vi "Actor Core.vi"(8 "error in":errorcluster, 11 "Nested in":refnum<class "UI_Top.lvclass">) -> (0 "error out":errorcluster, 3 "Actor out":refnum<class "Actor.lvclass">)   [LabVIEW 2021, in "UI_Top.lvclass"]
doc: "(<B>Filename</B>: Actor Framework.lvlib:Actor.lvclass:Actor Core.vi)\n\nReceives messages to the actor, reacts to them, and initiates any error handling that may shut the actor down.\n\nDescendant classes may override this VI to append parallel tasks for the actor to complete while it handles messages. Overrides use the Call Parent Method node."
uses:
  UI_Top.lvclass
  C:/Program Files (x86)/National Instruments/LabVIEW 2021/user.lib/John_Lib/AbstractActorTemplate/AbstractActorTemplate/UIActorTop.lvclass
  C:/Program Files (x86)/National Instruments/LabVIEW 2021/vi.lib/ActorFramework/Actor/Actor.lvclass
  <vilib>/ActorFramework/Actor/Actor.lvclass
  <userlib>/John_Lib/Control/Panel State.ctl
  UI_Top.lvclass/UI_Top.ctl
  <vilib>/ActorFramework/Actor/Actor.lvclass/Actor.ctl
  <vilib>/ActorFramework/Message Enqueuer/Message Enqueuer.lvclass/Message Enqueuer.ctl
  <userlib>/John_Lib/AbstractActorTemplate/UIActorTop Messages/UI Front Panel State Msg/UI Front Panel State Msg.lvclass/UI Front Panel State Msg.ctl
  <vilib>/ActorFramework/Message Enqueuer/Init from Existing Queue.vi
  <vilib>/ActorFramework/Message Enqueuer/Enqueue.vi
  <userlib>/John_Lib/AbstractActorTemplate/UIActorTop Messages/UI Front Panel State Msg/UI Front Panel State Msg.lvclass
  C:/Program Files (x86)/National Instruments/LabVIEW 2021/vi.lib/ActorFramework/Message/Message.lvclass
  <vilib>/ActorFramework/Stop Msg/Stop Msg.lvclass
  <vilib>/ActorFramework/Message Priority Queue/Priority Enqueue.vi
  <vilib>/ActorFramework/Message Enqueuer/Message Enqueuer.lvclass
  <userlib>/John_Lib/AbstractActorTemplate/AbstractActorTemplate/UIActorTop.lvclass
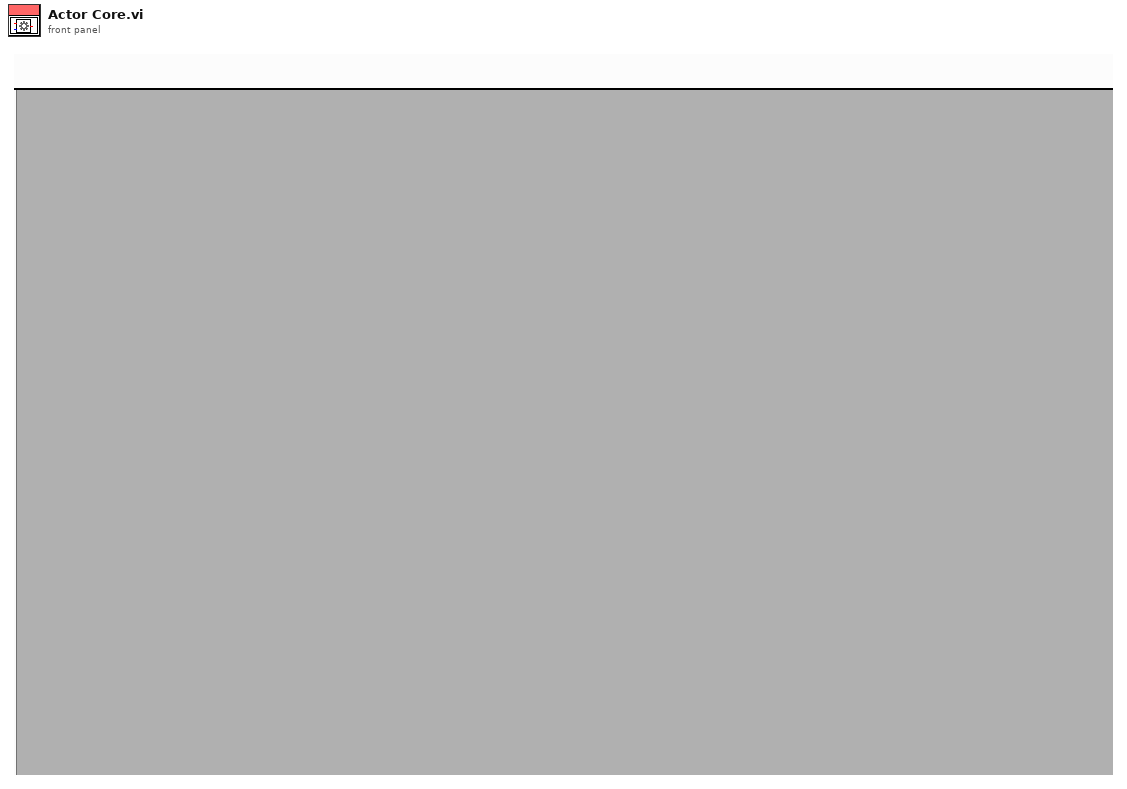
[diagram p1: front panel]
types:
  T1 = typedef "Panel State.ctl" = string
  T2 = typedef "sizeaction.ctl" = enum32{"Minimized", "Maximized", "Resized"}
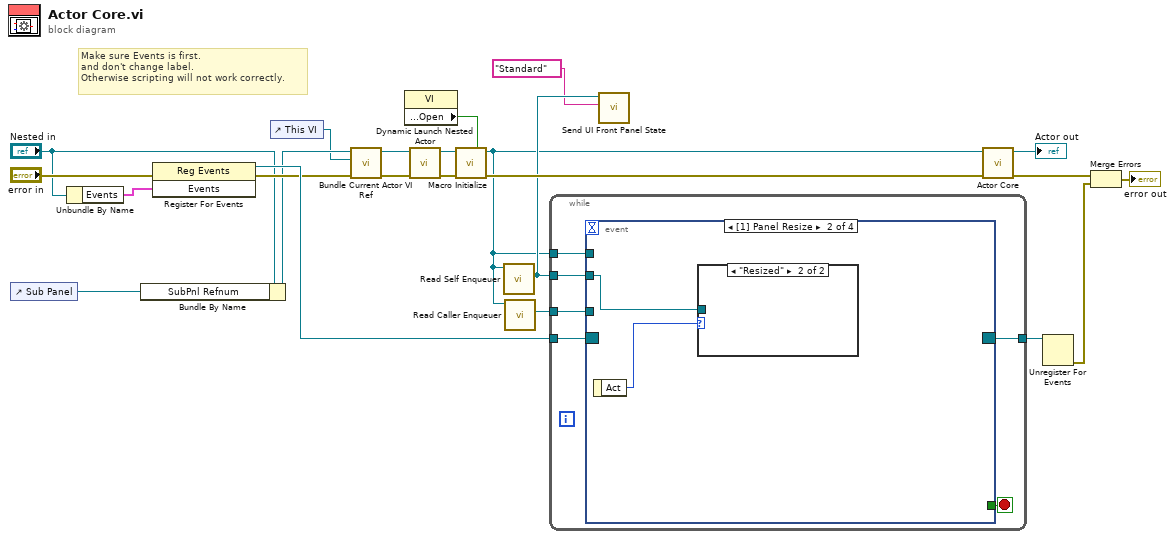
[diagram p0: block diagram]
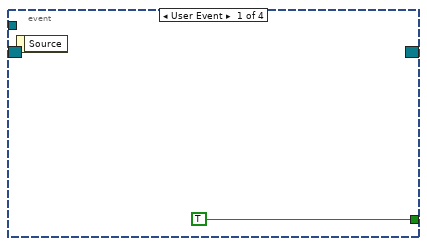
[diagram p2: hidden frame]
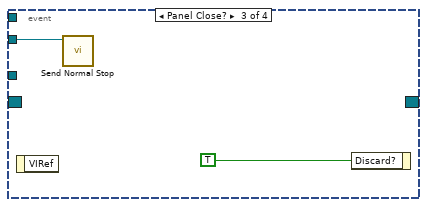
[diagram p4: hidden frame]
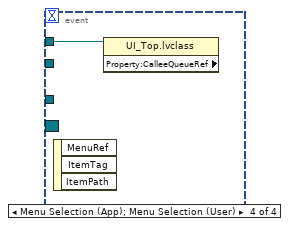
[diagram p5: hidden frame]
diagram:
  # "Make sure Events is first.\nand don't change label.\nOtherwise scripting will not work correctly."
  n1 = control-ref of="Sub Panel"() -> (w5:refnum<vi>)
  n2 = Unbundle By Name("Nested in") -> ("Events"=w21:cluster{"Stop":refnum<user-event>})
  n3 = Bundle By Name(cluster="Nested in", "SubPnl Refnum"=w5) -> (w6:refnum<class "UI_Top.lvclass">)
  n4 = register-events ("Main Register for Events")(error in="error in", w21) -> (reference out=w22:refnum<event-registration>, error out=w9:errorcluster)  [unwired: 1 in]
  n5 = control-ref of="This VI"() -> (w4:refnum<vi>)
  n6 = call <userlib>:"Bundle Current Actor VI Ref.vi"("error in (no error)"=w9, "This VI"=w4, "UI ActorTop in"=w6) -> ("error out"=w8:errorcluster, "UI ActorTop out"=w10:refnum<class "UI_Top.lvclass">)  [unwired: 5 in, 2 out]
  n7 = property class="VI"() -> ("Front Panel.Open"=w17:bool)  [unwired: 2 in, 2 out]
  n8 = call-dynamic "Dynamic Launch Nested Actor.vi"("error in (no error)"=w8, "UI ActorTop in"=w10) -> ("error out"=w18:errorcluster, "UI ActorTop out"=w19:refnum<class "UI_Top.lvclass">)  [unwired: 8 in]
  n9 = call-dynamic "Macro Initialize.vi"("Front Panel Window:Open"=w17, "error in (no error)"=w18, "UI ActorTop in"=w19) -> ("error out"=w12:errorcluster, "UI ActorTop out"=w2:refnum<class "UI_Top.lvclass">)  [unwired: 7 in]
  n10 = call <vilib>:"Read Self Enqueuer.vi"("Actor"=w2) -> ("Self Enqueuer"=w7:refnum<class "Message Enqueuer.lvclass">)  [unwired: 10 in]
  n11 = call <vilib>:"Read Caller Enqueuer.vi"("Actor"=w2) -> ("Caller Enqueuer"=w11:refnum<class "Message Enqueuer.lvclass">)  [unwired: 10 in]
  n12 = while {
    tunnel: w22 -> [w29]
    tunnel: [w27] -> w20
    tunnel: w7 -> [w26]
    tunnel: w11 -> [w25]
    tunnel: w2 -> [w24]
    stop <- w28 stop-if-true
    n13 = event "UI Events" shown="[1] Panel Resize" {
      selector: w29 -> [_ _ _ _]
      dyn-events: [_ _ _ _] -> w27
      timeout: _ -> [_ _ _ _]
      tunnel: [TRUE _ _ _] -> w28
      tunnel: w26 -> [_ w31 w33 _]
      tunnel: w25 -> [_ _ _ _]
      tunnel: w24 -> [_ _ _ w35]
      event User Event {
        n14 = event-data() -> ()  [unwired: 1 in, 1 out]
      }
      event Panel Resize {
        n15 = event-data() -> ("Act"=w32:T2)  [unwired: 1 in]
        n16 = case shown="\"Resized\"" w32 {
          tunnel: w31 -> [_ _]
          frame "Minimized", Default {
          }
          frame "Resized" {
          }
        }
      }
      event Panel Close? {
        n17 = event-data() -> ()  [unwired: 1 in, 1 out]
        n18 = call <vilib>:"Send Normal Stop.vi"("Message Enqueuer"=w33) -> ()  [unwired: 10 in, 1 out]
        n19 = event-data("Discard?"=TRUE) -> ()  [unwired: 1 in, 1 out]
      }
      event Menu Selection (App); Menu Selection (User) {
        n20 = event-data() -> ()  [unwired: 1 in, 3 out]
        n21 = property class="UI_Top.lvclass" props=["Property:CalleeQueueRef"](reference=w35) -> ()  [unwired: 1 in, 3 out]
      }
    }
  }
  n22 = call <userlib>:"Send UI Front Panel State.vi"("Argument"=T1 "Standard", "Message Enqueuer"=w7) -> ()  [unwired: 8 in, 2 out]
  n23 = call-parent "Actor Core.vi"("error in"=w12, "Actor in"=w2) -> ("error out"=w14:errorcluster, "Actor out"=→"Actor out":refnum<class "Actor.lvclass">)  [unwired: 8 in]
  n24 = Unregister For Events(event registration refnum=w20) -> (error out=w15:errorcluster)  [unwired: 1 in]
  n25 = Merge Errors(w14, w15) -> (→"error out":errorcluster)
